vi "Find peaks in file.vi"(8 "Error In":errorcluster, 9 "Channel names":string[](array[string])=["X", "Y", "Frequency"], 10 "group name":string="RUS160210180614", 11 "File Path Control":path=path "C:/Data/February_2016/020916/ms014_020916.tdms") -> (0 "Error Out":errorcluster)   [LabVIEW 2015]
panel:
  # "of max"
  # "Hz"
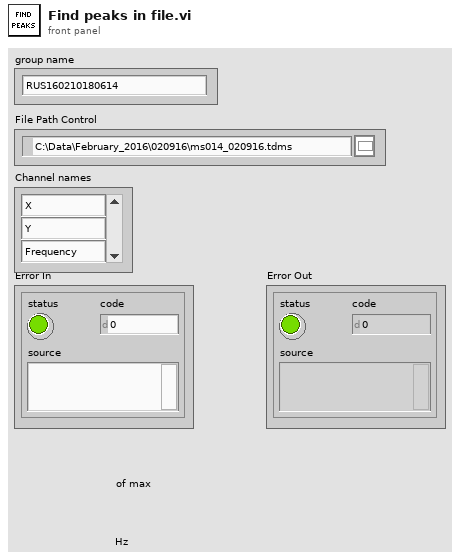
[diagram p1: front panel]
types:
  T1 = enum16{"open", "open or create", "create or replace", "create", "open (read-only)"}
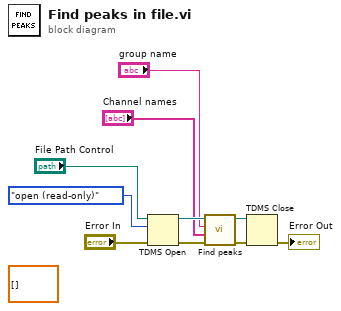
[diagram p0: block diagram]
diagram:
  (unwired) dbl[][] []
  n1 = TDMS Open(8:"Error In", 10:T1."open (read-only)" ("operation (0:open)"), 11:"File Path Control") -> (0:w3:errorcluster, 3:w6:refnum<k34>)  [unwired: 4 in]
  n2 = call "Find peaks.vi"("Error In"=w3, "Channel names"="Channel names", "group name"="group name", "tdms file"=w6) -> ("Error Out"=w4:errorcluster, "tdms file out"=w5:refnum<k34>)  [unwired: 3 in, 3 out]
  n3 = TDMS Close(8:w4, 11:w5) -> (0:→"Error Out":errorcluster)  [unwired: 1 out]
